vi "GT Get Follow Event.vi"(0 "cardNum":i16, 1 "pPos":i32, 5 "profile":i16, 7 "pEvent":i16, 9 "pMasterDir":i16, 11 "error in (no error)":errorcluster caption="错误输入（无错误）") -> (3 "pPos out":i32, 4 "function return":i16, 8 "pEvent out":i16, 10 "pMasterDir out":i16, 15 "error out":errorcluster caption="错误输出")   [LabVIEW 2014, in "gts.lvlib"]
doc: "GT_API GT_GetFollowEvent(short cardNum,short profile,short *pEvent,short *pMasterDir,long *pPos=NULL);"
uses:
  gts.lvlib
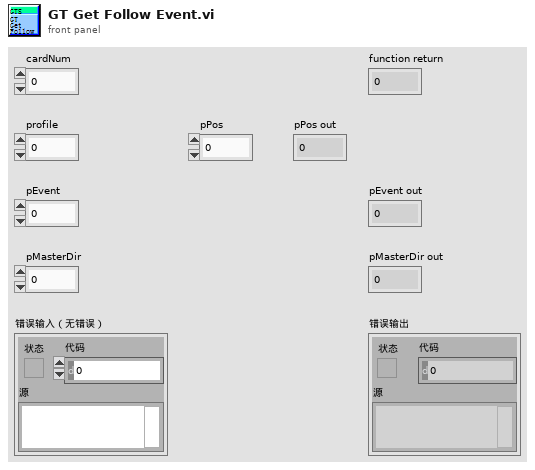
[diagram p1: front panel]
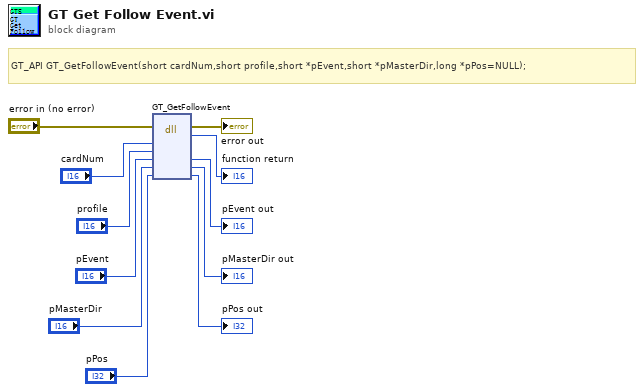
[diagram p0: block diagram]
diagram:
  # "GT_API GT_GetFollowEvent(short cardNum,short profile,short *pEvent,short *pMasterDir,long *pPos=NULL);"
  n1 = dll-call lib="PTH2habs D固高科技资料GTS控制卡GTS卡18年上半年资料dllVC32bit\nmulti_cardgts.*" fn="GT_GetFollowEvent"(error in="error in (no error)", "cardNum"="cardNum", "profile"="profile", "pEvent"="pEvent", "pMasterDir"="pMasterDir", "pPos"="pPos") -> (error out=→"error out":errorcluster, →"function return":i16, "pEvent"=→"pEvent out":i16, "pMasterDir"=→"pMasterDir out":i16, "pPos"=→"pPos out":i32)  [unwired: 4 in, 1 out]
